vi "SaveDeviceHeader.vi"(0 "File Refnum in":refnum<file>, 2 "no. of arrays":i32, 3 "Array Lengths":i32, 5 "Filename":string, 7 "RunNr":i32, 9 "Array Titles":string, 11 "error in (no error)":errorcluster, 12 "Temperature":dbl, 14 "Humidity":dbl) -> (4 "File Refnum out":refnum<file>, 6 "Header string":string, 15 "error out":errorcluster)   [LabVIEW 2018]
uses:
  globals/QC_RunInformation.vi
  globals/QC_MeasurementSetup.vi
  InstrControl/InstrumentSetup.vi
  InstrControl/SupplyControl/SupplyControl.lvclass
  InstrControl/LCRControl/LCRControl.lvclass
  InstrControl/InstrControl.lvclass
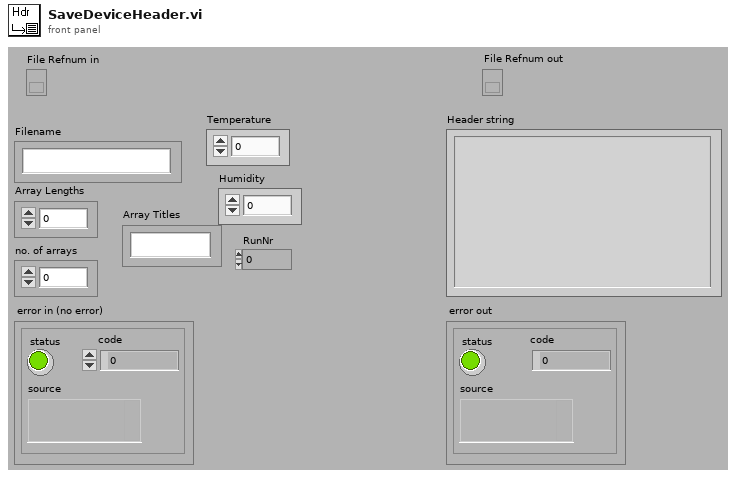
[diagram p1: front panel]
types:
  T1 = cluster{"RC Configuration":u16, "AC amplitude [V]":dbl, "AC frequency [Hz]":i32, "WK6440B":refnum<class "WK6440B.lvclass">}
  T2 = cluster{"Bias Supply":refnum<class "SupplyControl.lvclass">, "SMU":refnum<class "SupplyControl.lvclass">, "LCR":refnum<class "LCRControl.lvclass">, "Probe Card Channels":i32, "Bias Voltage [V]":dbl, "First strip":i32, "Last strip":i32, "Base Voltage [V]":dbl, "Base Ramp Step [V]":dbl, "Base Ramp Interval [ms]":u32, "High Voltage [V]":dbl, "High Ramp Step [V]":dbl, "High Ramp Interval [ms]":u32, "Single Needle":bool, "Temperature Readout":enum16{"Read Arduino", "Enter manually"}, "Arduino":refnum<class "ArduinoControl.lvclass">, "Fraction of good strips [%]":dbl, "ProbeStation":refnum<class "ProbeStationControl.lvclass">, "AC frequency [Hz]":i32, "Switching":refnum<class "Switching.lvclass">, "Matrix used?":bool, "Matrix X Channels":cluster{"Bias Supply / SMU LO":i32, "Bias Supply / SMU HI":i32, "CV Box LO":i32, "CV Box HI":i32, "CV Box LO IN":i32, "CV Box HI IN":i32, "Volt meter LO":i32, "Volt meter HI":i32, "Mux1 C1":i32, "Mux1 C2":i32, "Mux2 C1":i32, "Mux2 C2":i32}, "Pinholes Y/N":bool, "Capacitance Y/N":bool, "Resistance Y/N":bool}
  T3 = cluster{"Sensor Serial No.:":string, "Wafer Serial No.:":string, "Batch:":string, "Manufacturer:":string, "Device Category:":string, "Database Serial No.:":string, "Initiated:":string, "Test":string, "Instruments used:":string, "Probeplan used:":string, "End of Run comment:":string, "User:":string}
  T4 = cluster{"Institute":string, "Manufacturers":string[], "Devices":string[], "Serialnumbers Lookup DB":string, "Data directory":string, "Backup & screenshot directory":string, "List of known users":string[]}
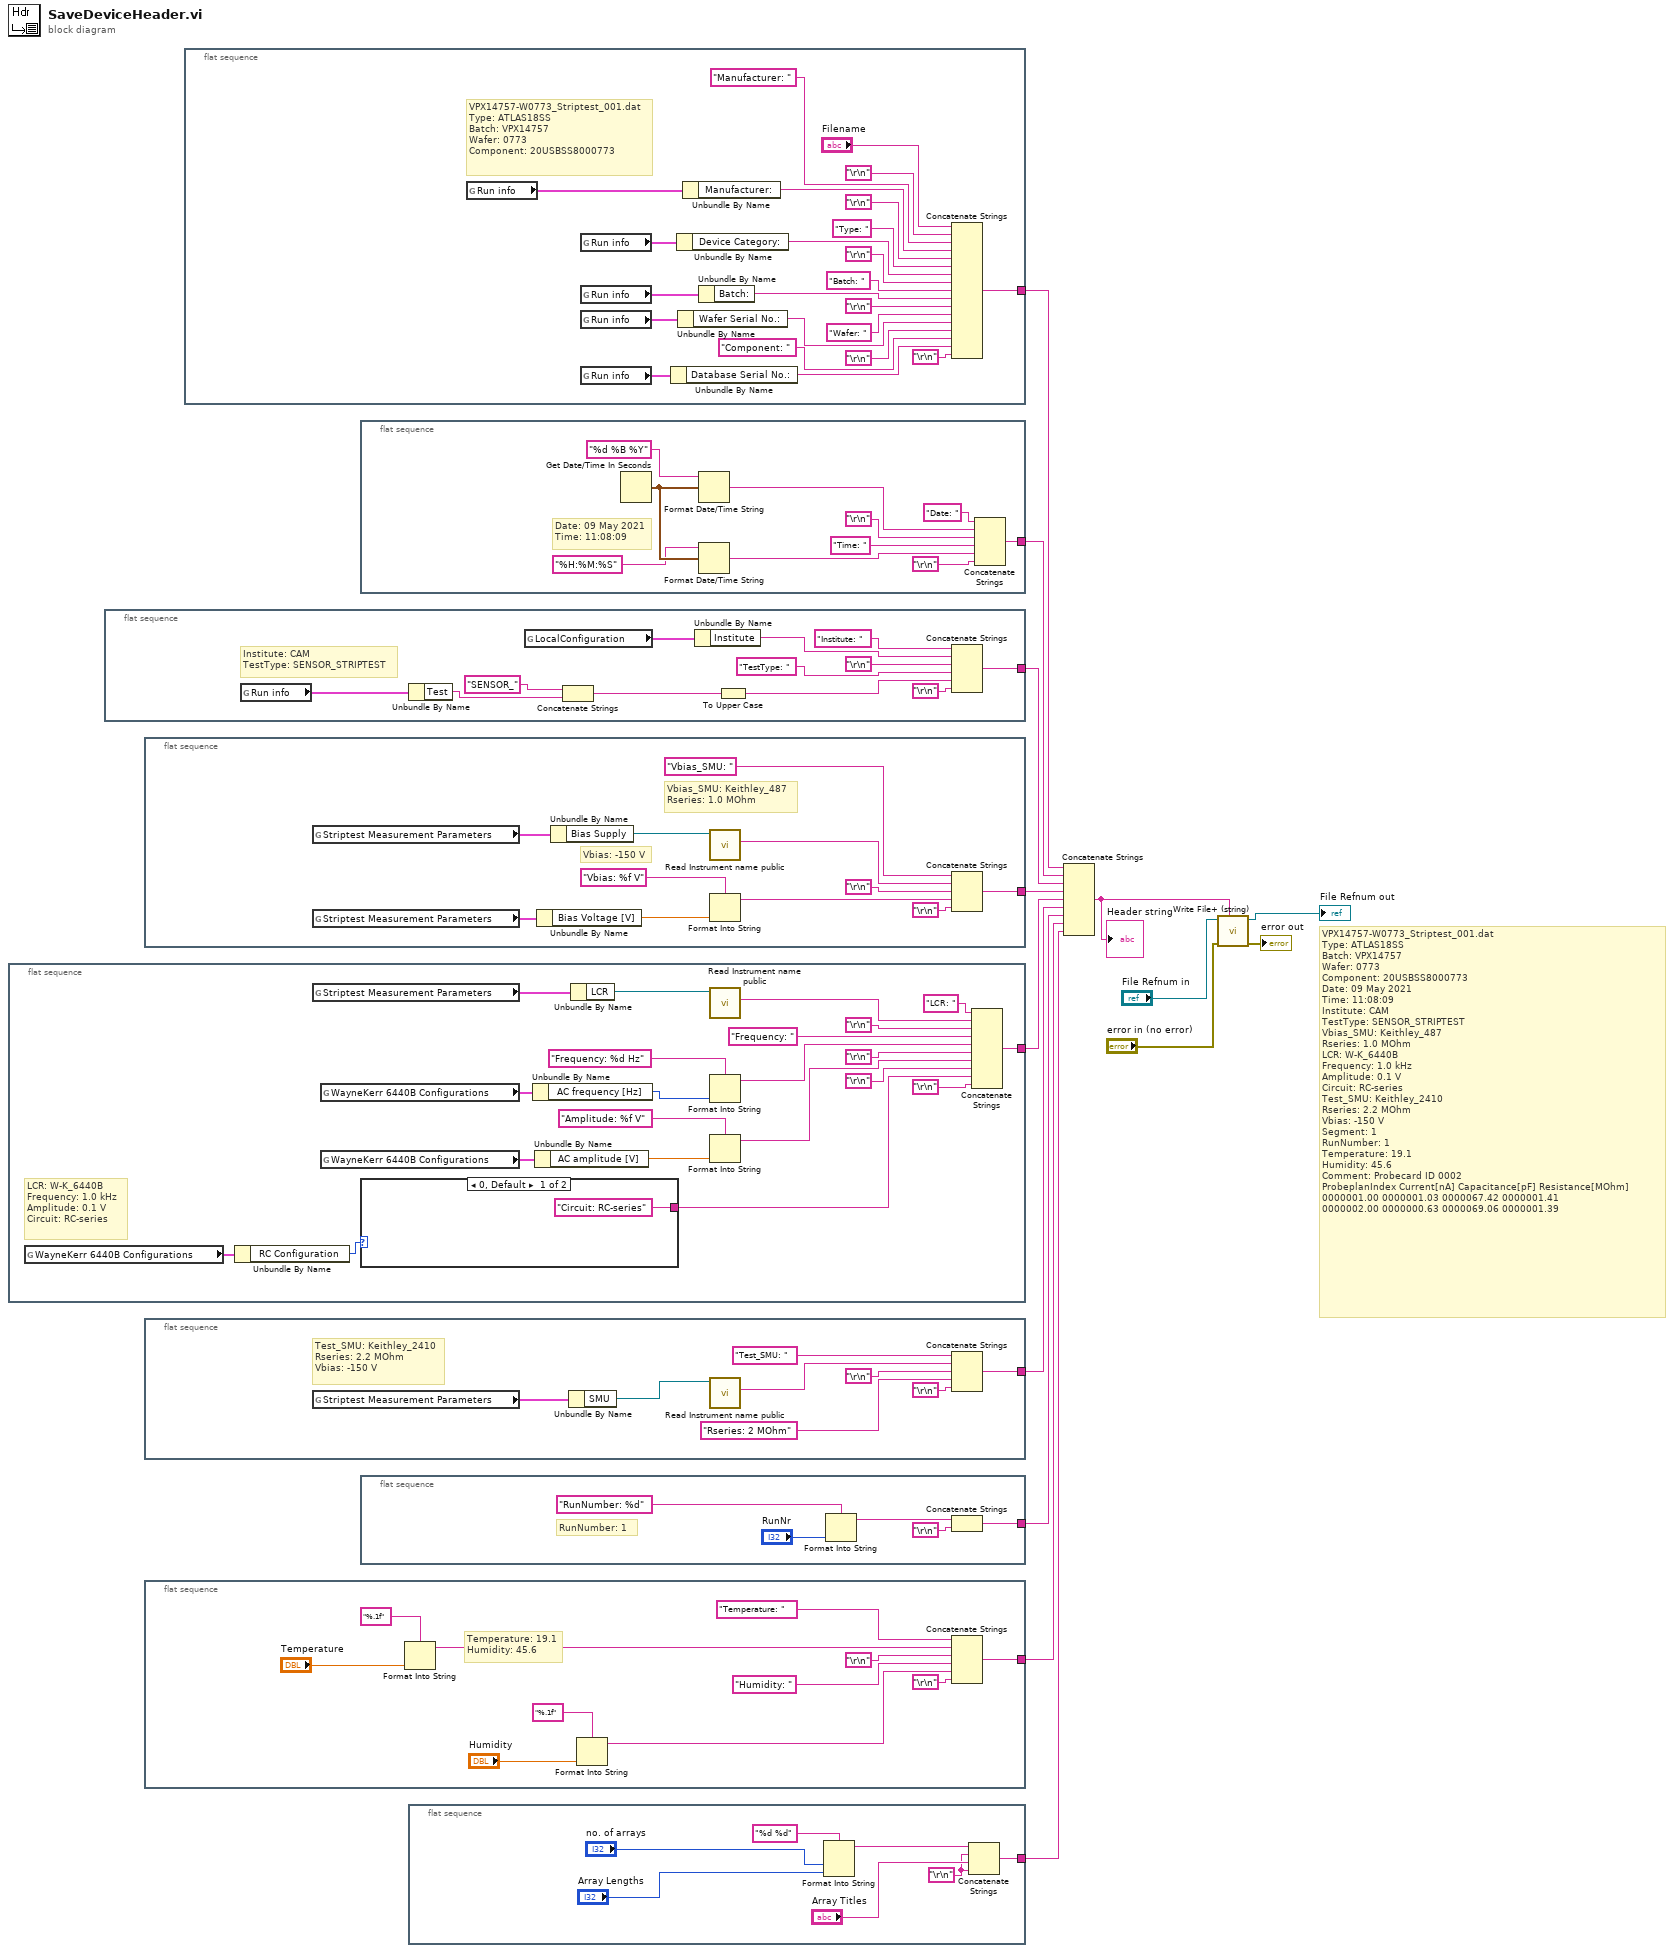
[diagram p0: block diagram]
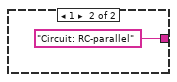
[diagram p2: hidden frame]
diagram:
  # "VPX14757-W0773_Striptest_001.dat\nType: ATLAS18SS\nBatch: VPX14757\nWafer: 0773\nComponent: 20USBSS8000773\nDate: 09 May 2021\nTime: 11:08:09\nInstitute: CAM\nTestType: SENSOR_STRIPTEST\nVbias_SMU: Keithley_487\nRseries: 1.0 MOhm\nLCR: W-K_6440B\nFrequency: 1.0 kHz\nAmplitude: 0.1 V\nCircuit: RC-series\nTest_SMU: Keithley_2410\nRseries: 2.2 MOhm\nVbias: -150 V\nSegment: 1\nRunNumber: 1\nTemperature: 19.1\nHumidity: 45.6\nComment: Probecard ID 0002\nProbeplanIndex Current[nA] Capacitance[pF] Resistance[MOhm]\n0000001.00 0000001.03 0000067.42 0000001.41\n0000002.00 0000000.63 0000069.06 0000001.39"
  n1 = flat-sequence {
    tunnel: [w17] -> w3
    frame #0 {
      # "LCR: W-K_6440B\nFrequency: 1.0 kHz\nAmplitude: 0.1 V\nCircuit: RC-series"
      n2 = global read "InstrumentSetup.vi" "WayneKerr 6440B Configurations"() -> (w21:T1)
      n3 = Unbundle By Name(w21) -> ("RC Configuration"=w20:u16)
      n4 = global read "QC_MeasurementSetup.vi" "Striptest Measurement Parameters"() -> (w33:T2)
      n5 = global read "InstrumentSetup.vi" "WayneKerr 6440B Configurations"() -> (w29:T1)
      n6 = global read "InstrumentSetup.vi" "WayneKerr 6440B Configurations"() -> (w28:T1)
      n7 = case shown="0, Default" w20 {
        tunnel: ["Circuit: RC-series" ("string") "Circuit: RC-parallel" ("string")] -> w19
        frame 0, Default {
        }
        frame 1 {
        }
      }
      n8 = Unbundle By Name(w29) -> ("AC frequency [Hz]"=w23:i32)
      n9 = Unbundle By Name(w28) -> ("AC amplitude [V]"=w26:dbl)
      n10 = Unbundle By Name(w33) -> ("LCR"=w16:refnum<class "LCRControl.lvclass">)
      n11 = call-dynamic "Read Instrument name public.vi"("InstrControl in"=w16) -> ("Instrument name"=w15:string)  [unwired: 8 in, 2 out]
      n12 = Format Into String(format string="Frequency: %d Hz", w23) -> (resulting string=w22:string)  [unwired: 2 in, 1 out]
      n13 = Format Into String(format string="Amplitude: %f V", w26) -> (resulting string=w25:string)  [unwired: 2 in, 1 out]
      n14 = Concatenate Strings("LCR: " ("string"), w15, "\r\n", "Frequency: " ("string"), w22, "\r\n", w25, "\r\n", w19, "\r\n") -> (w17:string)
    }
  }
  n15 = flat-sequence {
    tunnel: [w38] -> w8
    frame #0 {
      # "Institute: CAM\nTestType: SENSOR_STRIPTEST"
      n16 = global read "QC_RunInformation.vi" "Run info"() -> (w47:T3)
      n17 = Unbundle By Name(w47) -> ("Test"=w48:string)
      n18 = global read "QC_RunInformation.vi" "LocalConfiguration"() -> (w45:T4)
      n19 = Concatenate Strings("SENSOR_" ("string"), w48) -> (w49:string)
      n20 = Unbundle By Name(w45) -> ("Institute"=w43:string)
      n21 = To Upper Case(1:w49) -> (0:w39:string)
      n22 = Concatenate Strings("Institute: " ("string"), w43, "\r\n", "TestType: " ("string"), w39, "\r\n") -> (w38:string)
    }
  }
  n23 = flat-sequence {
    tunnel: [w52] -> w4
    frame #0 {
      # "Vbias: -150 V"
      # "Vbias_SMU: Keithley_487\nRseries: 1.0 MOhm"
      n24 = global read "QC_MeasurementSetup.vi" "Striptest Measurement Parameters"() -> (w60:T2)
      n25 = global read "QC_MeasurementSetup.vi" "Striptest Measurement Parameters"() -> (w56:T2)
      n26 = Unbundle By Name(w56) -> ("Bias Voltage [V]"=w55:dbl)
      n27 = Unbundle By Name(w60) -> ("Bias Supply"=w50:refnum<class "SupplyControl.lvclass">)
      n28 = call-dynamic "Read Instrument name public.vi"("InstrControl in"=w50) -> ("Instrument name"=w51:string)  [unwired: 8 in, 2 out]
      n29 = Format Into String(format string="Vbias: %f V", w55) -> (resulting string=w54:string)  [unwired: 2 in, 1 out]
      n30 = Concatenate Strings("Vbias_SMU: " ("string"), w51, "\r\n", w54, "\r\n") -> (w52:string)
    }
  }
  n31 = flat-sequence {
    tunnel: [w63] -> w2
    frame #0 {
      # "Test_SMU: Keithley_2410\nRseries: 2.2 MOhm\nVbias: -150 V"
      n32 = global read "QC_MeasurementSetup.vi" "Striptest Measurement Parameters"() -> (w66:T2)
      n33 = Unbundle By Name(w66) -> ("SMU"=w62:refnum<class "SupplyControl.lvclass">)
      n34 = call-dynamic "Read Instrument name public.vi"("InstrControl in"=w62) -> ("Instrument name"=w61:string)  [unwired: 8 in, 2 out]
      n35 = Concatenate Strings("Test_SMU: " ("string"), w61, "\r\n", "Rseries: 2 MOhm" ("string"), "\r\n") -> (w63:string)
    }
  }
  n36 = flat-sequence {
    tunnel: [w69] -> w6
    frame #0 {
      # "Temperature: 19.1\nHumidity: 45.6"
      n37 = Format Into String(format string="%.1f", "Temperature") -> (resulting string=w76:string)  [unwired: 2 in, 1 out]
      n38 = Format Into String(format string="%.1f", "Humidity") -> (resulting string=w71:string)  [unwired: 2 in, 1 out]
      n39 = Concatenate Strings("Temperature: " ("string"), w76, "\r\n", "Humidity: " ("string"), w71, "\r\n") -> (w69:string)
    }
  }
  n40 = flat-sequence {
    tunnel: [w87] -> w10
    frame #0 {
      # "VPX14757-W0773_Striptest_001.dat\nType: ATLAS18SS\nBatch: VPX14757\nWafer: 0773\nComponent: 20USBSS8000773"
      n41 = global read "QC_RunInformation.vi" "Run info"() -> (w86:T3)
      n42 = global read "QC_RunInformation.vi" "Run info"() -> (w99:T3)
      n43 = global read "QC_RunInformation.vi" "Run info"() -> (w98:T3)
      n44 = global read "QC_RunInformation.vi" "Run info"() -> (w97:T3)
      n45 = global read "QC_RunInformation.vi" "Run info"() -> (w101:T3)
      n46 = Unbundle By Name(w101) -> ("Database Serial No.:"=w102:string)
      n47 = Unbundle By Name(w99) -> ("Device Category:"=w94:string)
      n48 = Unbundle By Name(w97) -> ("Wafer Serial No.:"=w96:string)
      n49 = Unbundle By Name(w86) -> ("Manufacturer:"=w85:string)
      n50 = Unbundle By Name(w98) -> ("Batch:"=w95:string)
      n51 = Concatenate Strings("Filename", "\r\n", "Manufacturer: " ("string"), w85, "\r\n", "Type: " ("string"), w94, "\r\n", "Batch: " ("string"), w95, "\r\n", "Wafer: " ("string"), w96, "\r\n", "Component: " ("string"), w102, "\r\n") -> (w87:string)
    }
  }
  n52 = flat-sequence {
    tunnel: [w103] -> w9
    frame #0 {
      # "Date: 09 May 2021\nTime: 11:08:09"
      n53 = Get Date/Time In Seconds() -> (seconds since 1Jan1904=w112:timestamp)
      n54 = Format Date/Time String(time format string (%c)="%d %B %Y", seconds (now)=w112) -> (date/time string=w108:string)  [unwired: 1 in]
      n55 = Format Date/Time String(time format string (%c)="%H:%M:%S", seconds (now)=w112) -> (date/time string=w104:string)  [unwired: 1 in]
      n56 = Concatenate Strings("Date: " ("string"), w108, "\r\n", "Time: " ("string"), w104, "\r\n") -> (w103:string)
    }
  }
  n57 = flat-sequence {
    tunnel: [w114] -> w7
    frame #0 {
      # "RunNumber: 1"
      n58 = Format Into String(format string="RunNumber: %d" ("string"), "RunNr") -> (resulting string=w115:string)  [unwired: 2 in, 1 out]
      n59 = Concatenate Strings(w115, "\r\n") -> (w114:string)
    }
  }
  n60 = flat-sequence {
    tunnel: [w118] -> w5
    frame #0 {
      w119 = "\r\n"
      n61 = Format Into String(format string="%d %d", "no. of arrays", "Array Lengths") -> (resulting string=w122:string)  [unwired: 2 in, 1 out]
      n62 = Concatenate Strings(w122, w119, "Array Titles", w119) -> (w118:string)
    }
  }
  n63 = Concatenate Strings(w10, w9, w8, w4, w3, w2, w7, w6, w5) -> (w1:string)
  "Header string" <- w1
  n64 = call <vilib>:"Write File+ (string).vi"("string"=w1, "error in (no error)"="error in (no error)", "refnum"="File Refnum in") -> ("error out"=→"error out":errorcluster, "dup refnum"=→"File Refnum out":refnum<file>)  [unwired: 4 in, 1 out]
